vi "Get AO StringsAndValues.vi"(8 "error in (no error)":errorcluster, 11 "Configuration.DAQ":T1 {"AI.Coupling" items=["AC"=10045, "DC"=10050, "GND"=10066]}) -> (0 "error out":errorcluster, 2 "AO Strings and Values":cluster{string, i32}[](array[cluster]))   [LabVIEW 2019, in "Instrument UI.Lockin.lvclass"]
uses:
  Instrument UI.Lockin.lvclass
  Instrument.DAQ/Typedefs/DAQ.Configuration--Cluster--Array.ctl
  Instrument.DAQ/Typedefs/DAQ.Configuration--Cluster.ctl
  Instrument.DAQ/Typedefs/DAQ.Config.AO.Range--enum.ctl
  Instrument.DAQ/Typedefs/DAQ.Config.AI.Range--enum.ctl
  Instrument.DAQ/Typedefs/DAQ.Config.AI.Coupling--enum.ctl
  Instrument.DAQ/Instrument.DAQ.lvclass
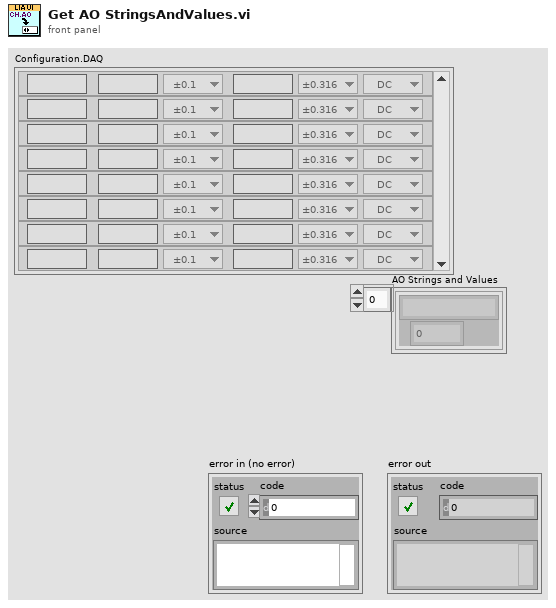
[diagram p1: front panel]
types:
  T1 = typedef "Instrument.DAQ.lvclass/DAQ.Configuration--Cluster--Array.ctl" = T2[]
  T2 = typedef "Instrument.DAQ.lvclass/DAQ.Configuration--Cluster.ctl" = cluster{"Device":string, "AO.Ch":string, "AO.Range":T3, "AI.Ch":string, "AI.Range":T4, "AI.Coupling":T5}
  T3 = typedef "Instrument.DAQ.lvclass/DAQ.Config.AO.Range--enum.ctl" = enum16{"±0.1", "±1.0", "±10.0"}
  T4 = typedef "Instrument.DAQ.lvclass/DAQ.Config.AI.Range--enum.ctl" = enum16{"±0.316", "±1.00", "±3.16", "±10.0", "±31.6", "±42.4"}
  T5 = typedef "Instrument.DAQ.lvclass/DAQ.Config.AI.Coupling--enum.ctl" = u16
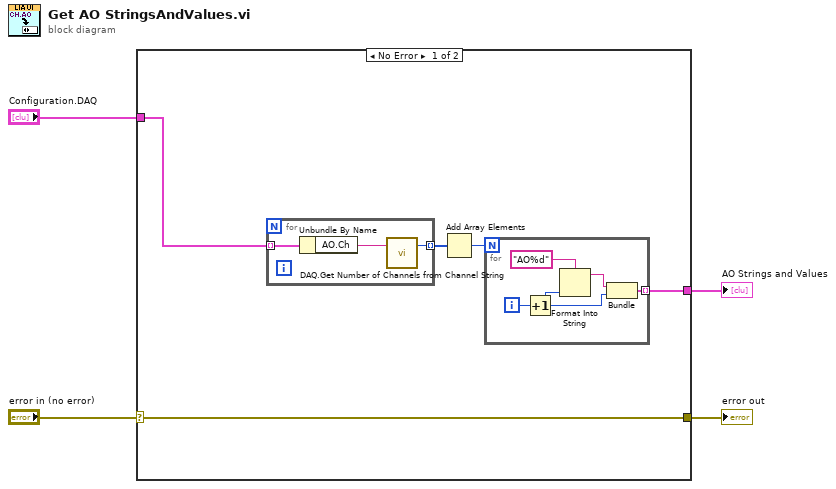
[diagram p0: block diagram]
diagram:
  n1 = case shown="No Error" "error in (no error)" {
    selector: "error in (no error)" -> [w6 w18]
    tunnel: "Configuration.DAQ" -> [w5 _]
    tunnel: [w7 _] -> w3
    tunnel: [w6 w18] -> w1
    frame No Error {
      n2 = for {
        tunnel: w5 -> [w12] mode=indexing
        tunnel: [w11] -> w8 mode=indexing
        n3 = Unbundle By Name(w12) -> ("AO.Ch"=w10:string)
        n4 = call "DAQ.Get Number of Channels from Channel String.vi"("Channels String"=w10) -> ("# channels"=w11:i32)  [unwired: 2 in]
      }
      n5 = Add Array Elements(numeric array=w8) -> (sum=w9:i32)
      n6 = for {
        N: w9 -> [_]
        tunnel: [w16] -> w7 mode=indexing
        i -> [w17]
        n7 = Increment(x=w17) -> (x+1=w15:i32)
        n8 = Format Into String(format string="AO%d", w15) -> (resulting string=w13:string)  [unwired: 2 in, 1 out]
        n9 = Bundle(w13, w15) -> (w16:cluster{string, i32})  [unwired: 1 in]
      }
    }
    frame Error {
    }
  }
  "AO Strings and Values" <- w3
  "error out" <- w1
